vi "set_output_type.vi"(8 "error in (no error)":errorcluster, 9 "output type":u8, 10 "output number":u8, 11 "VISA resource name":refnum<visa-resource-name>) -> (0 "error out":errorcluster, 3 "VISA resource name out":refnum<visa-resource-name>)   [LabVIEW 2018, in "Inficon IC6.lvlib"]
doc: "Update the type of an output.\n\nOutputs can be normally open or normally closed."
uses:
  <instrlib>/Inficon IC6/Inficon IC6.lvlib
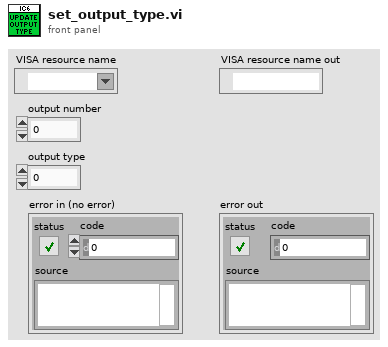
[diagram p1: front panel]
types:
  T1 = enum16{"Source", "General", "Input name", "Process name", "Logic", "Material", "Material name", "Output name", "Process", "Sensor", "Output type", "User message", "Layer", ""}
  T2 = enum16{"Hello", "Query", "Remote action", "Status", "Update"}
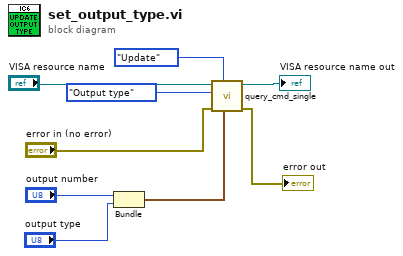
[diagram p0: block diagram]
diagram:
  n1 = Bundle("output number"="output number", "output type"="output type") -> (w3:cluster{"output number":u8, "output type":u8})  [unwired: 1 in]
  n2 = call <instrlib>:"query_cmd_single.vi"("Parameter"=w3, "Command group"=T2."Update", "error in (no error)"="error in (no error)", "Command subgroup"=T1."Output type", "VISA resource name"="VISA resource name") -> ("error out"=→"error out":errorcluster, "VISA resource name out"=→"VISA resource name out":refnum<visa-resource-name>)  [unwired: 2 in, 3 out]
